vi "Test Using Label.vi"(11 "Test Case In":refnum<class "Basic Mechanics Tests.lvclass">) -> (0 "error out":errorcluster, 3 "Test Case Out":refnum<class "Basic Mechanics Tests.lvclass">)   [LabVIEW 2020, in "Basic Mechanics Tests.lvclass"]
uses:
  Basic Mechanics Tests.lvclass
  C:/Program Files/National Instruments/LabVIEW 2026/vi.lib/Astemes/LUnit/Test Case.lvclass
  Source/Approval Tests/Options/Options.lvclass
  Source/Approval Tests/Report Nothing/Report Nothing.lvclass
  C:/Users/SAS/Desktop/ApprovalTests.LabVIEW/Source/Approval Tests/Reporter/Reporter.lvclass
  <vilib>/Astemes/LUnit/Test Case.lvclass/Test Case.ctl
  Source/Approval Tests/Options/Options.lvclass/Options.ctl
  Source/Approval Tests/Naming Data/Naming Data.lvclass/Naming Data.ctl
  7c504455-4432-4103-815a-1e4e68436cf8.vi
  00cd8e1e-9294-4dfd-9449-bcfe6af9dae2.vi
  228cf4e6-3bb9-4389-871e-800a2b29e1bd.vi
  Source/Approval Tests/Options/Write Reporter.vi
  <vilib>/Astemes/LUnit/Core/LUnit Test Case/Private/Append Pass Result.vi
  <vilib>/Astemes/LUnit/Core/LUnit Test Case/Private/Append Fail Result.vi
  Source/Approval Tests/Verify Core.vi
  7c504455-4432-4103-815a-1e4e68436cf8.vi/93c5622b-9fb7-41e0-8c76-3fde37e94e34.vi
  Source/Approval Tests/Options/Update Test Name if Not Defined.vi
  Source/Approval Tests/Options/Read Scrubber.vi
  00cd8e1e-9294-4dfd-9449-bcfe6af9dae2.vi/9c5d11cd-9439-4240-a1ee-d9baace9c924.vi
  228cf4e6-3bb9-4389-871e-800a2b29e1bd.vi/9c5d11cd-9439-4240-a1ee-d9baace9c924.vi
  <vilib>/Astemes/LUnit/Core/LUnit Test Case/Private/Run In UI.vi
  Source/Approval Tests/Options/Read Namer.vi
  Source/Approval Tests/Options/Read Naming Data.vi
  Source/Approval Tests/Options/Read Reporter.vi
  Source/Approval Tests/Options/Read Text Comparator.vi
  7c504455-4432-4103-815a-1e4e68436cf8.vi/93c5622b-9fb7-41e0-8c76-3fde37e94e34.vi/04cb982b-2eda-40d0-8d7e-90f8e0b569b2.vi
  Source/Approval Tests/Naming Data/Read Test VI Name.vi
  Source/Approval Tests/Naming Data/Write Test VI Name.vi
  Source/Approval Tests/Options/Add Label to Namer.vi
  Source/Approval Tests/conv EOL.vi
  Source/Approval Tests/Reporter/Report.vi
  Source/Approval Tests/Scrubber/Scrubber.lvclass
  Source/Approval Tests/Namer/Namer.lvclass
  Source/Approval Tests/Naming Data/Naming Data.lvclass
  Source/Approval Tests/Reporter/Reporter.lvclass
  Source/Approval Tests/Text Comparator/Text Comparator.lvclass
  <vilib>/Astemes/LUnit/Test Case.lvclass
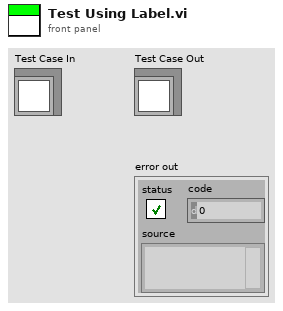
[diagram p1: front panel]
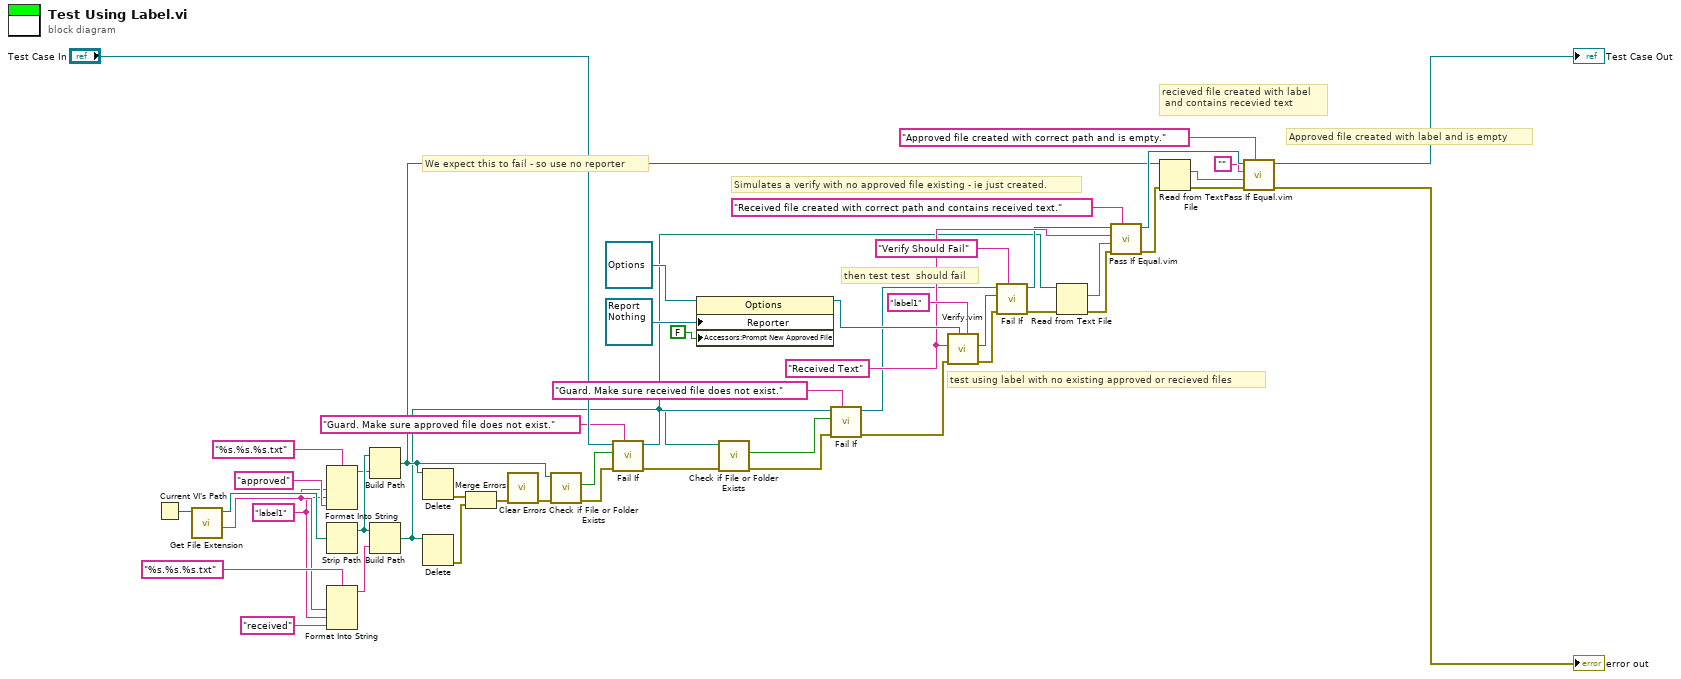
[diagram p0: block diagram]
diagram:
  w28 = "label1" ("input 2")
  w18 = "Received Text"
  # "Approved file created with label and is empty"
  # "recieved file created with label\n and contains recevied text"
  # "then test test  should fail"
  # "test using label with no existing approved or recieved files"
  # "We expect this to fail - so use no reporter"
  # "Simulates a verify with no approved file existing - ie just created."
  n1 = Current VI's Path() -> (path=w36:path)
  n2 = call <vilib>:"Get File Extension.vi"("file"=w36) -> ("filename without extension"=w29:string, "dup file"=w35:path)  [unwired: 6 in, 3 out]
  n3 = Format Into String(format string="%s.%s.%s.txt", w29, w28, "approved" ("string")) -> (resulting string=w30:string)  [unwired: 2 in, 1 out]
  n4 = Strip Path(path=w35) -> (stripped path=w34:path)  [unwired: 1 out]
  n5 = Format Into String(format string="%s.%s.%s.txt", w29, w28, "received" ("string")) -> (resulting string=w26:string)  [unwired: 2 in, 1 out]
  n6 = Build Path(base path=w34, name or relative path=w30) -> (appended path=w9:path)
  n7 = Build Path(base path=w34, name or relative path=w26) -> (appended path=w3:path)
  n8 = Delete(path (use dialog)=w9) -> (error out=w42:errorcluster)  [unwired: 4 in, 2 out]
  n9 = Delete(path (use dialog)=w3) -> (error out=w47:errorcluster)  [unwired: 4 in, 2 out]
  n10 = Merge Errors(w42, w47) -> (w46:errorcluster)
  n11 = call <vilib>:"Clear Errors.vi"("error in (no error)"=w46) -> ("error out"=w39:errorcluster)  [unwired: 5 in, 1 out]
  n12 = call <vilib>:"Check if File or Folder Exists.vi"("error in (no error)"=w39, "path"=w9) -> ("error out"=w40:errorcluster, "file or folder exists?"=w6:bool)  [unwired: 7 in, 1 out]
  n13 = call <vilib>:"Fail If.vi"("Description"="Guard. Make sure approved file does not exist.", "error in (no error)"=w40, "Fail?"=w6, "LUnit Test Case In"="Test Case In") -> ("error out"=w41:errorcluster, "LUnit Test Case Out"=w8:refnum<class "Basic Mechanics Tests.lvclass">)  [unwired: 6 in]
  n14 = property on="Property Node" class="Options"(reference=refnum<class "Options.lvclass"> refnum ("Options"), "Reporter"=refnum<class "Report Nothing.lvclass"> refnum ("Approval Tests.lvlib:Report Nothing"), "Accessors:Prompt New Approved File"=FALSE ("Prompt New Approved File")) -> (reference out=w23:refnum<class "Options.lvclass">)  [unwired: 1 in, 1 out]
  n15 = call <vilib>:"Check if File or Folder Exists.vi"("error in (no error)"=w41, "path"=w3) -> ("error out"=w37:errorcluster, "file or folder exists?"=w2:bool)  [unwired: 7 in, 1 out]
  n16 = call <vilib>:"Fail If.vi"("Description"="Guard. Make sure received file does not exist.", "error in (no error)"=w37, "Fail?"=w2, "LUnit Test Case In"=w8) -> ("error out"=w38:errorcluster, "LUnit Test Case Out"=w7:refnum<class "Basic Mechanics Tests.lvclass">)  [unwired: 6 in]
  n17 = call "Verify.vim"("Label"="label1", "Options"=w23, "error in"=w38, "Anything"=w18) -> ("error out"=w50:errorcluster, "Passed?"=w15:bool)  [unwired: 5 in, 1 out]
  n18 = call <vilib>:"Fail If.vi"("Description"="Verify Should Fail", "error in (no error)"=w50, "Fail?"=w15, "LUnit Test Case In"=w7) -> ("error out"=w43:errorcluster, "LUnit Test Case Out"=w16:refnum<class "Basic Mechanics Tests.lvclass">)  [unwired: 6 in]
  n19 = Read from Text File(file (use dialog)=w3, error in=w43) -> (text=w17:string, error out=w49:errorcluster)  [unwired: 2 in, 2 out]
  n20 = call "Pass If Equal.vim"("Description"="Received file created with correct path and contains received text.", "error in (no error)"=w49, "Actual"=w17, "Expected"=w18, "LUnit Test Case In"=w16) -> ("error out"=w44:errorcluster, "LUnit Test Case Out"=w19:refnum<class "Basic Mechanics Tests.lvclass">)  [unwired: 5 in]
  n21 = Read from Text File(file (use dialog)=w9, error in=w44) -> (text=w20:string, error out=w48:errorcluster)  [unwired: 2 in, 2 out]
  n22 = call "Pass If Equal.vim"("Description"="Approved file created with correct path and is empty.", "error in (no error)"=w48, "Actual"=w20, "Expected"="", "LUnit Test Case In"=w19) -> ("error out"=→"error out":errorcluster, "LUnit Test Case Out"=→"Test Case Out":refnum<class "Basic Mechanics Tests.lvclass">)  [unwired: 5 in]
